vi "SRV_Create 12-Char Timestamp.vi"(7 "sec since 01/01/1904 (-1: now)":dbl=-1.0 format="%.3f") -> (8 "Timestamp String":string)   [LabVIEW 2014]
doc: "Creates a timestamp string of the format:\nYYMMDDhhmmss\n\nLeave the input unwired to get the current timestamp.\n\n\nAuthor: Mike Schultz"
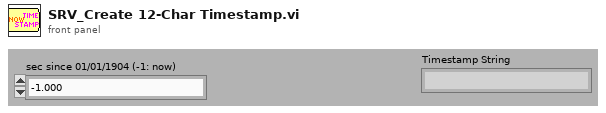
[diagram p1: front panel]
types:
  T1 = typedef "LVDateTimeRec.ctl" = cluster{"fractional second":dbl, "second":i32, "minute":i32, "hour":i32, "day of month":i32, "month":i32, "year":i32, "day of week":i32, "day of year":i32, "DST":i32}
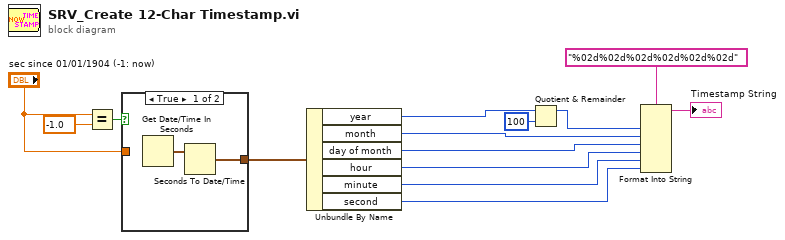
[diagram p0: block diagram]
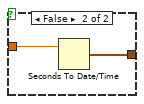
[diagram p2: hidden frame]
diagram:
  n1 = Equal?(x="sec since 01/01/1904 (-1: now)", y=-1.0) -> (x = y?=w8:bool)
  n2 = case shown="True" w8 {
    tunnel: [w15 w17] -> w14
    tunnel: "sec since 01/01/1904 (-1: now)" -> [_ w18]
    frame True {
      n3 = Get Date/Time In Seconds() -> (seconds since 1Jan1904=w16:timestamp)
      n4 = Seconds To Date/Time(time stamp (now)=w16) -> (date time rec=w15:T1)  [unwired: 1 out]
    }
    frame False {
      n5 = Seconds To Date/Time(time stamp (now)=w18) -> (date time rec=w17:T1)  [unwired: 1 out]
    }
  }
  n6 = Unbundle By Name(w14) -> ("year"=w9:i32, "month"=w4:i32, "day of month"=w3:i32, "hour"=w2:i32, "minute"=w1:i32, "second"=w13:i32)
  n7 = Quotient & Remainder(x=w9, y=100) -> (x-y*floor(x/y)=w10:i32)  [unwired: 1 out]
  n8 = Format Into String(format string="%02d%02d%02d%02d%02d%02d", w10, w4, w3, w2, w1, w13) -> (resulting string=→"Timestamp String":string)  [unwired: 2 in, 1 out]
